vi "Launch Root.vi"(5 "Status Q":refnum<class "MessageQ.lvclass">, 7 "VolatusAPI":refnum<class "VolatusAPI.lvclass">, 8 "error in (no error)":errorcluster, 9 "Config Element":refnum<class "VolatusConfigElement.lvclass">, 11 "Module in":refnum<class "Module.lvclass">) -> (0 "error out":errorcluster, 2 "MessageQ":refnum<class "MessageQ.lvclass">)   [LabVIEW 2020, in "Volatus.lvlib" / "Module.lvclass"]
uses:
  Module.lvclass
  VolatusAPI/VolatusAPI.lvclass
  MessageQ/MessageQ.lvclass
  VolatusConfig/VolatusConfigElement/VolatusConfigElement.lvclass
  Module.lvclass/Module.ctl
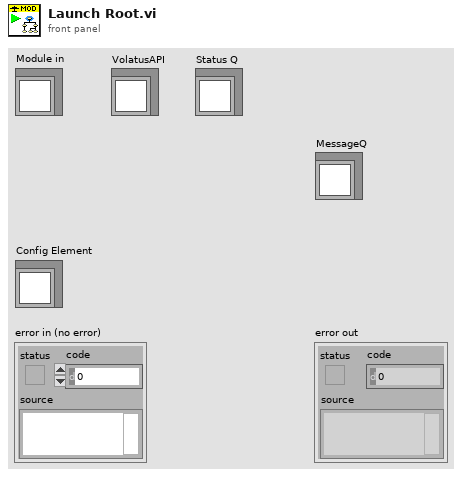
[diagram p1: front panel]
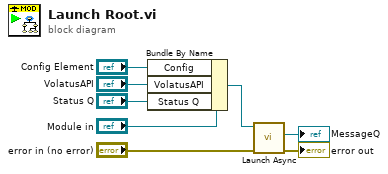
[diagram p0: block diagram]
diagram:
  n1 = Bundle By Name(cluster="Module in", "Config"="Config Element", "VolatusAPI"="VolatusAPI", "Status Q"="Status Q") -> (w6:refnum<class "Module.lvclass">)
  n2 = call "Launch Async.vi"("error in (no error)"="error in (no error)", "Module in"=w6) -> ("error out"=→"error out":errorcluster, "MessageQ"=→"MessageQ":refnum<class "MessageQ.lvclass">)  [unwired: 8 in]
